vi "testNetworkServerClient.vi"() -> ()   [LabVIEW 2009, in "run.lvlib"]
uses:
  testing/run.lvlib
  CameraNetworkClient/CameraNetworkServer.lvclass
  Channels/Camera/Camera/Camera.lvclass
  NetworkClient/NetworkServer.lvclass
  Tools/Filing/FileNeologist/FileNeologist.lvclass
panel:
  out "Remote connection":string
  in  "stop":bool
  # "Camera Server"
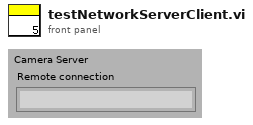
[diagram p1: front panel]
types:
  T1 = cluster{"Message":enum16{"Idle", "initialise", "configureAcquisition", "setTemperature", "getTemperature", "start", "stop", "sendImage", "close", "error", "ExitApp"}, "Data":variant}
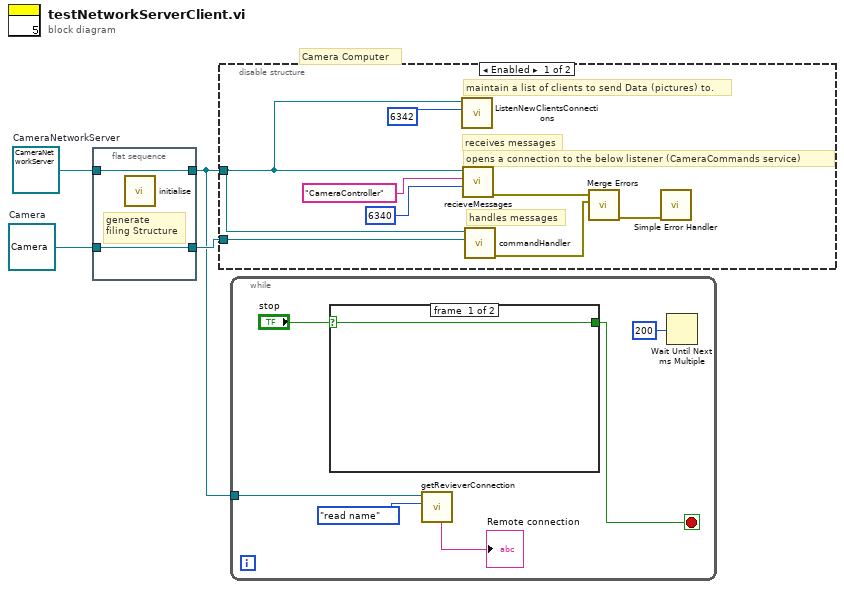
[diagram p0: block diagram]
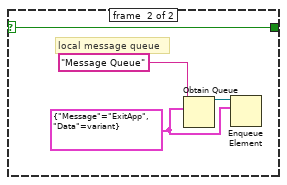
[diagram p2: hidden frame]
diagram:
  w2 = refnum<class "Camera.lvclass"> refnum  # Camera
  w4 = refnum<class "CameraNetworkServer.lvclass"> refnum  # CameraNetworkServer
  # "Camera Computer"
  n1 = flat-sequence {
    tunnel: [w6] -> w1
    tunnel: w4 -> [w6]
    tunnel: [w5] -> w3
    tunnel: w2 -> [w5]
    frame #0 {
      # "generate\nfiling Structure"
      n2 = call "initialise.vi"() -> ()  [unwired: 10 in, 2 out]
    }
  }
  n3 = disable-structure shown="Enabled" {
    disable-tunnel: w3 -> [w10 _]
    disable-tunnel: w1 -> [w9 _]
    frame #0 {
      # "maintain a list of clients to send Data (pictures) to."
      # "opens a connection to the below listener (CameraCommands service)"
      # "handles messages"
      # "receives messages"
      n4 = call "ListenNewClientsConnections.vi"("Port"=6342, "NetworkClient in"=w9) -> ()  [unwired: 8 in, 2 out]
      n5 = call "recieveMessages.vi"("port"=6340, "Service"="CameraController", "NetworkClient in"=w9) -> ("error out"=w14:errorcluster)  [unwired: 7 in, 1 out]
      n6 = call-dynamic "commandHandler.vi"("Camera"=w10, "CameraNetworkClient in"=w9) -> ("error out"=w13:errorcluster)  [unwired: 8 in, 1 out]
      n7 = call <vilib>:"Merge Errors.vi"("error in 2 (no error)"=w13, "error in 1 (no error)"=w14) -> ("error out"=w12:errorcluster)  [unwired: 5 in]
      n8 = call <vilib>:"Simple Error Handler.vi"("error in (no error)"=w12) -> ()  [unwired: 4 in, 5 out]
    }
    frame #1 {
    }
  }
  n9 = while {
    tunnel: w1 -> [w17]
    stop <- w19 stop-if-true
    n10 = case shown="True" "stop" {
      selector: "stop" -> [w21 w24]
      tunnel: [w21 w24] -> w19
      frame #0 {
      }
      frame #1 {
        w22 = T1 {"Message"=enum."ExitApp", "Data"=variant}
        # "local message queue"
        n11 = Obtain Queue(name (unnamed)="Message Queue" ("Queue Name"), element data type=w22) -> (queue out=w23:refnum<queue>)  [unwired: 3 in, 2 out]
        n12 = Enqueue Element(queue=w23, element=w22) -> ()  [unwired: 2 in, 3 out]
      }
    }
    n13 = call "getRevieverConnection.vi"("Enum"=enum16{"read", "write", "reset", "read name"}."read name", "NetworkServer in"=w17) -> ("Remote Connection"=→"Remote connection":string)  [unwired: 5 in, 4 out]
    n14 = Wait Until Next ms Multiple(millisecond multiple=200) -> ()  [unwired: 1 out]
  }
